vi "save_txt.vi"(8 "x":i32, 9 "z":i32, 10 "Data":dbl[][](array[numeric]) format="%0.2f", 11 "base path":path) -> ()   [LabVIEW 2016]
uses:
  <vilib>/Utility/file.llb/Write To Spreadsheet File (DBL).vi
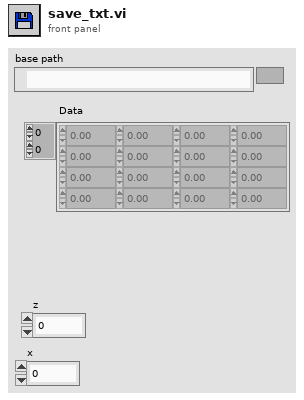
[diagram p1: front panel]
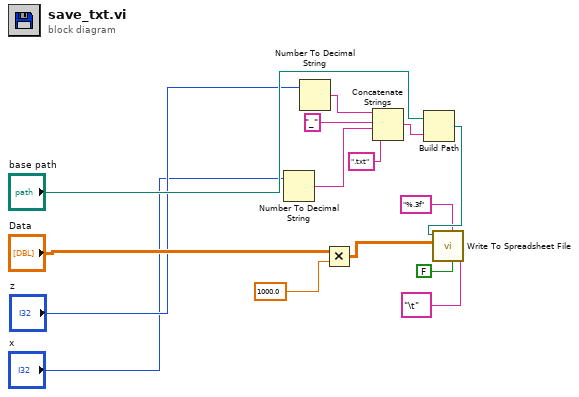
[diagram p0: block diagram]
diagram:
  n1 = Number To Decimal String(number="x") -> (decimal integer string=w11:string)  [unwired: 1 in]
  n2 = Number To Decimal String(number="z") -> (decimal integer string=w15:string)  [unwired: 1 in]
  n3 = Multiply(x="Data", y=1000.0) -> (x*y=w4:dbl[][])
  n4 = Concatenate Strings(w15, "_" ("string"), w11, ".txt" ("string")) -> (w13:string)
  n5 = Build Path(base path="base path", name or relative path=w13) -> (appended path=w12:path)
  n6 = call-poly <vilib>:"Write To Spreadsheet File.vi"("delimiter (\\t)"="\t", "transpose? (no:F)"=FALSE, "format (%.3f)"="%.3f", "2D data"=w4, "file path (dialog if empty)"=w12) -> ()  [unwired: 3 in, 1 out]
